vi "Hysteresis_max.vi"(0 "input(+)":dbl, 5 "input (-)":dbl, 7 "H":dbl=22.0 format="%#_13g", 9 "Max":dbl=26.0 format="%#_13g", 11 "error in":errorcluster) -> (8 "Deviation":bool, 15 "error out":errorcluster)   [LabVIEW 2022 SP3]
uses:
  MD_modules/MD420/MD420.lvclass/MD420.ctl
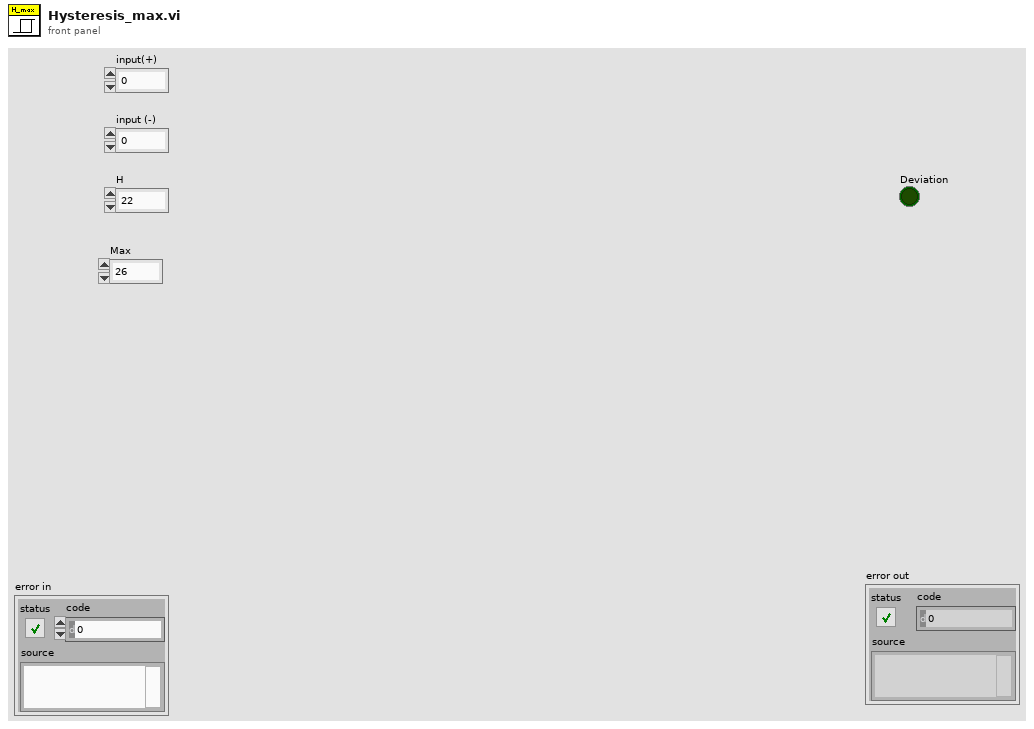
[diagram p1: front panel]
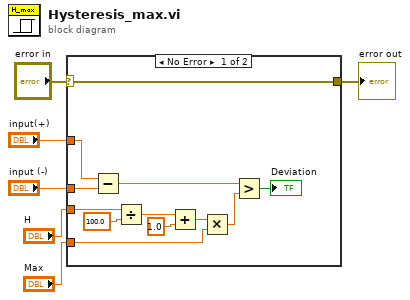
[diagram p0: block diagram]
diagram:
  n1 = case shown="No Error" "error in" {
    selector: "error in" -> [w11 w19]
    tunnel: [w11 w19] -> w5
    tunnel: "input(+)" -> [w10 _]
    tunnel: "input (-)" -> [w9 _]
    tunnel: "H" -> [w8 _]
    tunnel: "Max" -> [w7 _]
    frame No Error {
      n2 = Subtract(x=w10, y=w9) -> (x-y=w13:dbl)
      n3 = Divide(x=w8, y=100.0) -> (x/y=w14:dbl)
      n4 = Add(x=w14, y=1.0) -> (x+y=w16:dbl)
      n5 = Multiply(x=w16, y=w7) -> (x*y=w17:dbl)
      n6 = Greater?(x=w13, y=w17) -> (0:→"Deviation":bool)
    }
    frame Error {
    }
  }
  "error out" <- w5
